vi "Create Time string.vi"(8 "error in (no error)":errorcluster) -> (0 "error out":errorcluster, 3 "Timestr":string)   [LabVIEW 2018, in "Application.lvlib"]
uses:
  Application.lvlib
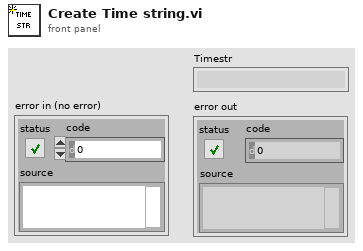
[diagram p1: front panel]
types:
  T1 = typedef "LVDateTimeRec.ctl" = cluster{"fractional second":dbl, "second":i32, "minute":i32, "hour":i32, "day of month":i32, "month":i32, "year":i32, "day of week":i32, "day of year":i32, "DST":i32}
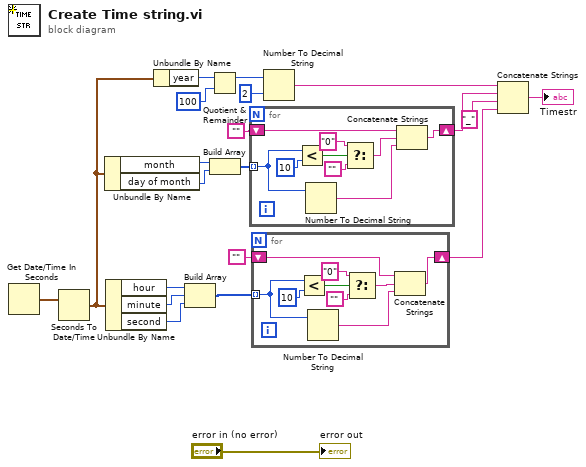
[diagram p0: block diagram]
diagram:
  n1 = Get Date/Time In Seconds() -> (seconds since 1Jan1904=w2:timestamp)
  n2 = Seconds To Date/Time(time stamp (now)=w2) -> (date time rec=w14:T1)  [unwired: 1 in]
  n3 = Unbundle By Name(w14) -> ("month"=w13:i32, "day of month"=w1:i32)
  n4 = Unbundle By Name(w14) -> ("hour"=w10:i32, "minute"=w9:i32, "second"=w8:i32)
  n5 = Unbundle By Name(w14) -> ("year"=w20:i32)
  n6 = Build Array(w10, w9, w8) -> (w7:i32[])
  n7 = Quotient & Remainder(x=w20, y=100) -> (x-y*floor(x/y)=w15:i32)  [unwired: 1 out]
  n8 = Build Array(w13, w1) -> (w12:i32[])
  n9 = for {
    tunnel: w12 -> [w24] mode=indexing
    shift-right: [w23] -> w6
    shift-left: "" -> [w22]
    n10 = Less?(x=w24, y=10) -> (x < y?=w29:bool)
    n11 = Number To Decimal String(number=w24) -> (decimal integer string=w25:string)  [unwired: 1 in]
    n12 = Select(t="0", s=w29, f="") -> (s? t:f=w26:string)
    n13 = Concatenate Strings(w22, w26, w25) -> (w23:string)
  }
  n14 = for {
    tunnel: w7 -> [w33] mode=indexing
    shift-right: [w32] -> w4
    shift-left: "" -> [w31]
    n15 = Less?(x=w33, y=10) -> (x < y?=w38:bool)
    n16 = Number To Decimal String(number=w33) -> (decimal integer string=w34:string)  [unwired: 1 in]
    n17 = Select(t="0", s=w38, f="") -> (s? t:f=w35:string)
    n18 = Concatenate Strings(w31, w35, w34) -> (w32:string)
  }
  n19 = Number To Decimal String(number=w15, width (-)=i16 2) -> (decimal integer string=w17:string)
  n20 = Concatenate Strings(w17, w6, "_" ("string"), w4) -> (→"Timestr":string)
  "error out" <- "error in (no error)"
